vi "SDKSID4_Camera GetAttribute.vi"(8 "error in (no error)":errorcluster, 10 "AttributeID":u16, 11 "SDKSID4 session In":T1) -> (0 "error out":errorcluster, 2 "AttributeValueOut":dbl, 3 "SDKSID4 session Out":T1)   [LabVIEW 2013]
doc: "This VI returns the current value of the camera attribute specified in input by its Attribute ID. The list of camera attributes and the associated ID are given by the \"Camera GetAttributeList\" function."
uses:
  Refnum SDKSID4 session.ctl
  SID4_SDK.dll
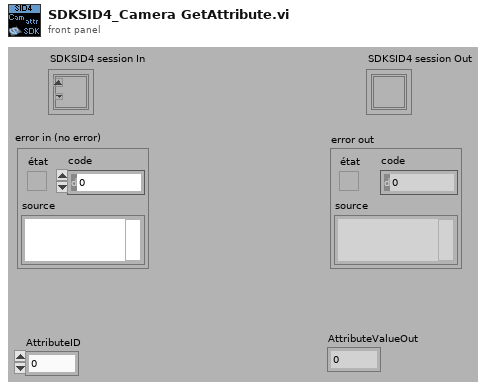
[diagram p1: front panel]
types:
  T1 = typedef "Refnum SDKSID4 session.ctl" = refnum<k1>
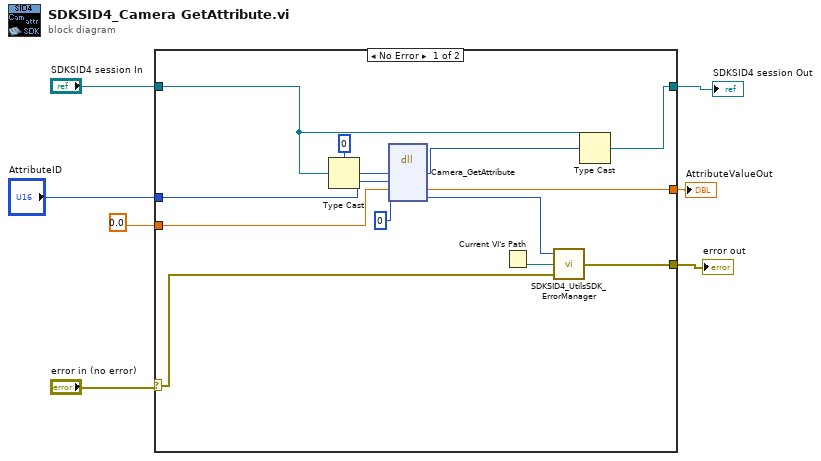
[diagram p0: block diagram]
diagram:
  n1 = case shown="No Error" "error in (no error)" {
    selector: "error in (no error)" -> [w13 w22]
    tunnel: "SDKSID4 session In" -> [w17 w23]
    tunnel: [w16 w23] -> w6
    tunnel: [w14 w22] -> w4
    tunnel: "AttributeID" -> [w12 _]
    tunnel: [w10 w21] -> w2
    tunnel: 0.0 -> [w9 w21]
    frame No Error {
      n2 = Type Cast(type=u32 0, x=w17) -> (*(type *) &x=w19:u32)
      n3 = dll-call lib="C:/Program Files/SID4_SDK/DLL SDK/BIN/SID4_SDK.dll" fn="Camera_GetAttribute"("SessionId"=w19, "AttributeID"=w12, "AttributeValueOut"=w9, "Error"=0) -> ("SessionId"=w18:u32, "AttributeValueOut"=w10:dbl, "Error"=w11:i32)  [unwired: 5 in, 2 out]
      n4 = Current VI's Path() -> (path=w15:path)
      n5 = call "SDKSID4_UtilsSDK_ErrorManager.vi"("error IN"=w13, "VI PathFile"=w15, "ErrorCode"=w11) -> ("error OUT"=w14:errorcluster)
      n6 = Type Cast(type=w17, x=w18) -> (*(type *) &x=w16:T1)
    }
    frame Error {
    }
  }
  "SDKSID4 session Out" <- w6
  "error out" <- w4
  "AttributeValueOut" <- w2
